vi "Start Output Items.vi"(8 "error in (no error)":errorcluster, 9 "Project In":refnum<class "Project.lvclass">, 10 "Output":T1[](array[typedef]), 11 "Item Panel in":refnum<vi>[](array[refnum])) -> (0 "error out":errorcluster, 1 "Output Item VI Ref":refnum<vi>[](array[refnum]), 3 "Item Panel out":refnum<vi>[](array[refnum]))   [LabVIEW 2015, in "OutputUI.lvclass"]
uses:
  OutputUI.lvclass
  Step/STEP_OUTPUT.ctl
  Step/OUTPUT_DATA_TYPE.ctl
  OUTPUT_CHECK_TYPE.ctl
  Step/OUTPUT_VALUE_TYPE.ctl
  Project.lvclass
  String/String Output Item.vi
  Numeric/Numeric Output Item.vi
  Other/Other Output Item.vi
  Step.lvclass
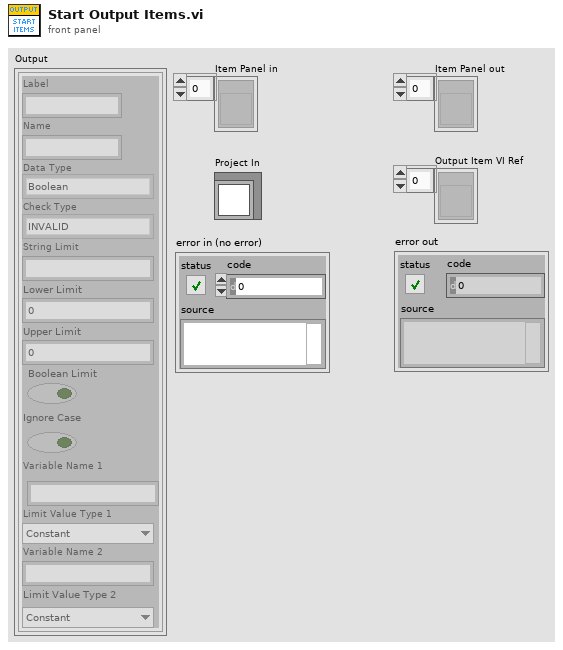
[diagram p1: front panel]
types:
  T1 = typedef "Step.lvclass/STEP_OUTPUT.ctl" = cluster{"Label":string, "Name":string, "Data Type":T2, "Check Type":T3, "String Limit":string, "Lower Limit":dbl, "Upper Limit":dbl, "Boolean Limit":bool, "Ignore Case":bool, "Variable Name 1":string, "Limit Value Type 1":T4, "Variable Name 2":string, "Limit Value Type 2":T4}
  T2 = typedef "Step.lvclass/OUTPUT_DATA_TYPE.ctl" = enum16{"Boolean", "String", "Numeric", "Other"}
  T3 = typedef "Step.lvclass/OUTPUT_CHECK_TYPE.ctl" = enum16{"INVALID", "DO_NOT_CHECK", "RECORD", "VARIABLE", "EQUAL", "NOT_EQUAL", "STR_CONTAINS", "STR_START_WITH", "STR_END_WITH", "STR_REGEX_MATCH", "NUM_GT", "NUM_LT", "NUM_GE", "NUM_LE", "NUM_RANGE", "NUM_RANGE_BDY"}
  T4 = typedef "Step.lvclass/OUTPUT_VALUE_TYPE.ctl" = enum16{"Constant", "Variable"}
  T5 = enum32{"Invalid", "Standard", "Closed", "Hidden", "Minimized", "Maximized"}
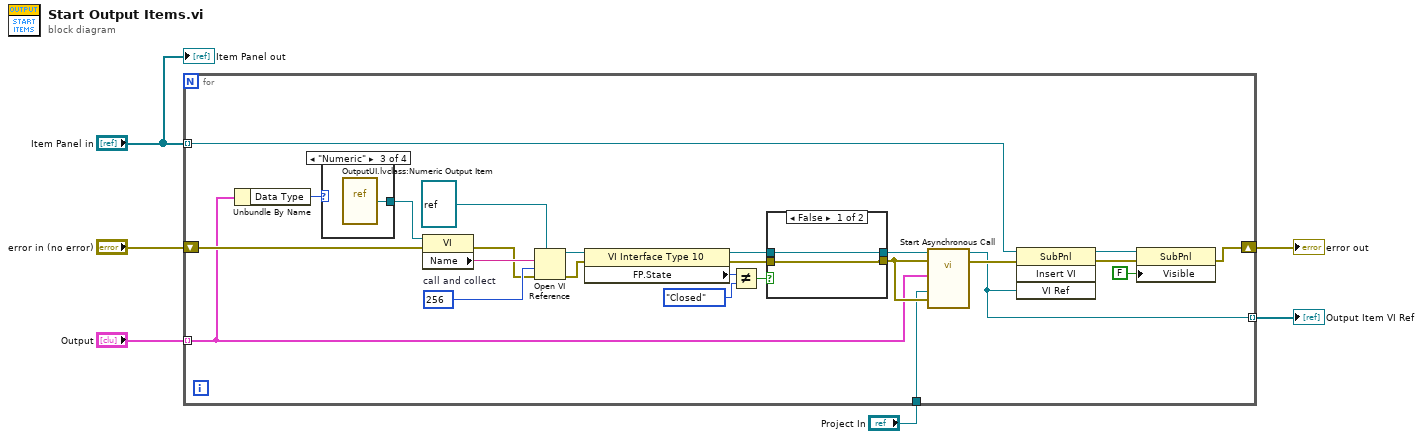
[diagram p0: block diagram]
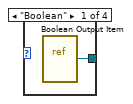
[diagram p2: hidden frame]
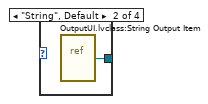
[diagram p3: hidden frame]
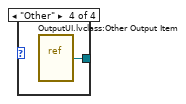
[diagram p4: hidden frame]
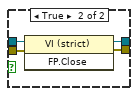
[diagram p5: hidden frame]
diagram:
  n1 = for {
    shift-right: [w11] -> w2
    shift-left: "error in (no error)" -> [w17]
    tunnel: "Output" -> [w8] mode=indexing
    tunnel: "Item Panel in" -> [w15] mode=indexing
    tunnel: [w14] -> w3 mode=indexing
    tunnel: "Project In" -> [w9]
    w28 = 256  # call and collect
    n2 = Unbundle By Name(w8) -> ("Data Type"=w7:T2)
    n3 = case shown="\"Numeric\"" w7 {
      tunnel: [w32 w33 w34 w35] -> w31
      frame "Boolean" {
        n4 = vi-ref "Boolean Output Item.vi"() -> (w32:refnum<vi>)
      }
      frame "String", Default {
        n5 = vi-ref "OutputUI.lvclass:String Output Item.vi"() -> (w33:refnum<vi>)
      }
      frame "Numeric" {
        n6 = vi-ref "OutputUI.lvclass:Numeric Output Item.vi"() -> (w34:refnum<vi>)
      }
      frame "Other" {
        n7 = vi-ref "OutputUI.lvclass:Other Output Item.vi"() -> (w35:refnum<vi>)
      }
    }
    n8 = property class="VI"(reference=w31, error in=w17) -> (error out=w27:errorcluster, "Name"=w29:string)  [unwired: 1 out]
    n9 = Open VI Reference(type specifier VI Refnum (for type only)=refnum<vi> refnum, vi path=w29, options=w28, error in (no error)=w27) -> (vi reference=w21:refnum<vi>, error out=w20:errorcluster)  [unwired: 2 in]
    n10 = property class="VI Interface Type 10"(reference=w21, error in=w20) -> (reference out=w25:refnum<vi>, error out=w26:errorcluster, "FP.State"=w22:T5)
    n11 = Not Equal?(x=w22, y=T5."Closed" ("Front Panel Window:State")) -> (x != y?=w24:bool)
    n12 = case shown="False" w24 {
      tunnel: w25 -> [w37 w41]
      tunnel: w26 -> [w36 w40]
      tunnel: [w37 w39] -> w19
      tunnel: [w36 w38] -> w18
      frame False {
      }
      frame True {
        n13 = invoke class="VI (strict)" method="FP.Close"(reference=w41, error in=w40) -> (reference out=w39:refnum<vi>, error out=w38:errorcluster)  [unwired: 1 in, 1 out]
      }
    }
    n14 = call-by-ref "Start Asynchronous Call"(reference=w19, error in=w18, 8:"error in (no error)"=w18, "Project In"=w9, "Output"=w8) -> (reference out=w14:refnum<vi>, error out=w16:errorcluster)  [unwired: 8 in, 1 out]
    n15 = invoke class="SubPnl" method="Insert VI"(reference=w15, error in=w16, "VI Ref"=w14) -> (reference out=w13:refnum<vi>, error out=w12:errorcluster)  [unwired: 1 in, 2 out]
    n16 = property class="SubPnl"(reference=w13, error in=w12, "Visible"=FALSE) -> (error out=w11:errorcluster)  [unwired: 1 out]
  }
  "error out" <- w2
  "Output Item VI Ref" <- w3
  "Item Panel out" <- "Item Panel in"
